vi "Step.GetProperties.vi"(11 "String in":string) -> (2 "Parameters":dbl[](array[numeric]), 3 "Step":T1)   [LabVIEW 2013, in "Simple Sequence Editor.lvlib"]
uses:
  Simple Sequence Editor.lvlib
  Types/StepTypes.ctl
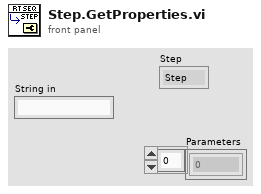
[diagram p1: front panel]
types:
  T1 = typedef "Simple Sequence Editor.lvlib/StepTypes.ctl" = enum8{"Step", "iStep", "Ramp", "Unchanged", "Unknown"}
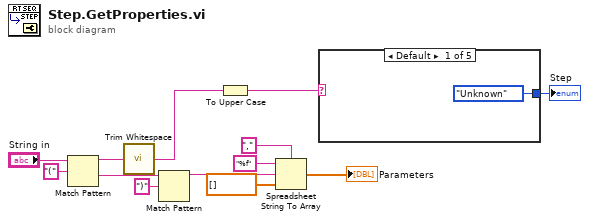
[diagram p0: block diagram]
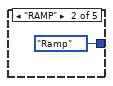
[diagram p2: hidden frame]
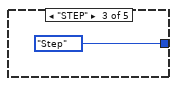
[diagram p3: hidden frame]
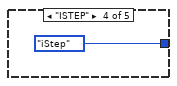
[diagram p4: hidden frame]
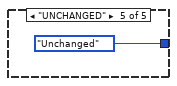
[diagram p5: hidden frame]
diagram:
  n1 = Match Pattern(string="String in", regular expression="(") -> (before substring=w5:string, after substring=w6:string)  [unwired: 1 in, 2 out]
  n2 = call <vilib>:"Trim Whitespace.vi"("string"=w5) -> ("trimmed string"=w12:string)  [unwired: 1 in]
  n3 = Match Pattern(string=w6, regular expression=")") -> (before substring=w8:string)  [unwired: 1 in, 3 out]
  n4 = To Upper Case(1:w12) -> (0:w2:string)
  n5 = Spreadsheet String To Array(delimiter (Tab)=",", format string="%f", spreadsheet string=w8, array type (2D Dbl)=dbl[] []) -> (array=→"Parameters":dbl[])
  n6 = case shown="Default" w2 {
    tunnel: [StepTypes."Unknown" StepTypes."Ramp" StepTypes."Step" StepTypes."iStep" StepTypes."Unchanged"] -> w1
    frame Default {
    }
    frame "RAMP" {
    }
    frame "STEP" {
    }
    frame "ISTEP" {
    }
    frame "UNCHANGED" {
    }
  }
  "Step" <- w1
